vi "Periodic Tasks.vi"(8 "error in":errorcluster) -> ()   [LabVIEW 2012]
doc: "This VI runs in parallel to other tasks. It can contain as many user-defined periodic loops as you need. These can carry out PID or other sorts of timed response."
uses:
  <vilib>/Rock Robotics/SystemInterfaces/Utilities/FPGA_UtilitiesLED Source.ctl
  <vilib>/Rock Robotics/SystemInterfaces/Utilities/FPGA_UtilitiesLED State.ctl
  <vilib>/Rock Robotics/WPI/Compressor/WPI_CompressorGetSetRefNum.vi
  Robot Global Data.vi
panel:
  out "Shooter Speed":dbl
  out "Shooter Distance":dbl
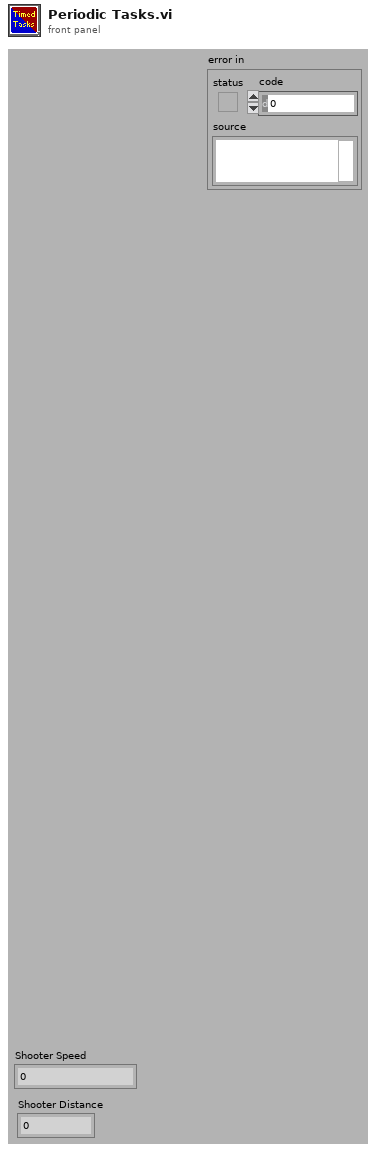
[diagram p1: front panel]
types:
  T1 = typedef "WPI_GyroDevRef.ctl" = cluster{"DevStatus":errorcluster, "Analog Module":T2, "Analog Channel":T3, "Offset":dbl, "Gain (VoltsPerDegree/Second)":dbl}
  T2 = typedef "FPGA_TypedefAnalogModule.ctl" = enum16{"Analog Module 1", "Analog Module 2"}
  T3 = typedef "FPGA_AIChannel.ctl" = enum8{"AI 1", "AI 2", "AI 3", "AI 4", "AI 5", "AI 6", "AI 7", "AI 8", "Invalid"}
  T4 = typedef "FPGA_UtilitiesLED State.ctl" = enum16{"Off", "On", "Toggle"}
  T5 = typedef "FPGA_UtilitiesLED Source.ctl" = enum16{"User LED", "FPGA LED"}
  T6 = typedef "WPI_DriverStationRobotMode2.ctl" = enum16{"Autonomous Disabled", "Autonomous Enabled", "Teleop Disabled", "Teleop Enabled", "Timeout", "Finish", "Test Disabled", "Test Enabled"}
  T7 = typedef "WPI_EncoderDevRef.ctl" = cluster{"DevStatus":errorcluster, "EncoderIndex":T8, "CounterIndex":T9, "DistancePerCount":dbl, "Decoding Type":T10}
  T8 = typedef "FPGA_EncoderIdx.ctl" = enum8{"Enc 0", "Enc 1", "Enc 2", "Enc 3", "Invalid"}
  T9 = typedef "FPGA_CounterCtrSystemIndex.ctl" = enum8{"Ctr 0", "Ctr 1", "Ctr 2", "Ctr 3", "Ctr 4", "Ctr 5", "Ctr 6", "Ctr 7", "Invalid"}
  T10 = typedef "WPI_EncoderType.ctl" = enum16{"1x", "2x", "4x"}
  T11 = enum16{"Off", "Close Pyramid 3pt", "Far Pyramid 3pt", "Feeder Shot", "UD Far 3pt Shot"}
  T12 = typedef "WPI_CompressorDevRef.ctl" = cluster{"DevStatus":errorcluster, "DigitalInputDevRef":T13, "RelayDevRef":T16}
  T13 = typedef "WPI_DigitalInputDevRef.ctl" = cluster{"DevStatus":errorcluster, "DIO Channel":T14, "Digital Module":T15}
  T14 = typedef "FPGA_DIOChannel.ctl" = enum8{"DIO 1", "DIO 2", "DIO 3", "DIO 4", "DIO 5", "DIO 6", "DIO 7", "DIO 8", "DIO 9", "DIO 10", "DIO 11", "DIO 12", "DIO 13", "DIO 14", "Invalid"}
  T15 = typedef "FPGA_TypedefDigitalModule.ctl" = enum16{"Digital Module 1", "Digital Module 2"}
  T16 = typedef "WPI_RelayDevRef.ctl" = cluster{"DevStatus":errorcluster, "Relay Channel":T17, "Digital Module":T15, "Relay Direction":T18}
  T17 = typedef "FPGA_DIORelayChannel.ctl" = enum8{"Relay 1", "Relay 2", "Relay 3", "Relay 4", "Relay 5", "Relay 6", "Relay 7", "Relay 8", "Invalid"}
  T18 = typedef "WPI_RelayDirection.ctl" = enum16{"Both directions", "Forward only", "Reverse only"}
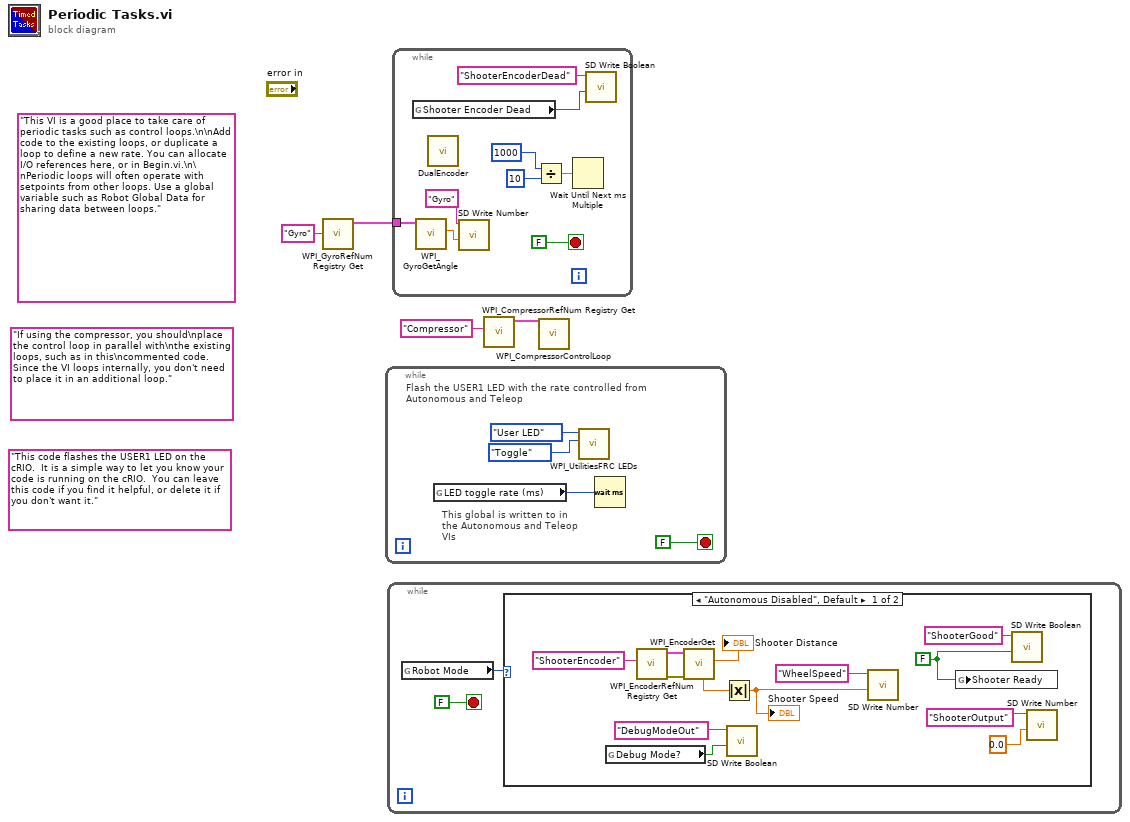
[diagram p0: block diagram]
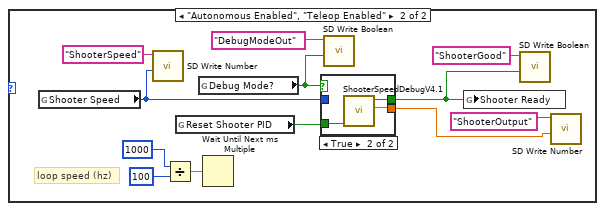
[diagram p2: hidden frame]
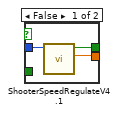
[diagram p3: hidden frame]
diagram:
  (unwired) "If using the compressor, you should\nplace the control loop in parallel with\nthe existing loops, such as in this\ncommented code. Since the VI loops internally, you don't need to place it in an additional loop."
  (unwired) "This code flashes the USER1 LED on the cRIO.  It is a simple way to let you know your code is running on the cRIO.  You can leave this code if you find it helpful, or delete it if you don't want it."
  (unwired) "This VI is a good place to take care of periodic tasks such as control loops.\n\nAdd code to the existing loops, or duplicate a loop to define a new rate. You can allocate I/O references here, or in Begin.vi.\n\nPeriodic loops will often operate with setpoints from other loops. Use a global variable such as Robot Global Data for sharing data between loops."
  n1 = call <vilib>:"WPI_GyroRefNum Registry Get.vi"("refnum name"="Gyro") -> ("GyroDevRef"=w3:T1)  [unwired: 9 in, 1 out]
  n2 = while {
    stop <- FALSE stop-if-true
    # "This global is written to in the Autonomous and Teleop VIs"
    # "Flash the USER1 LED with the rate controlled from Autonomous and Teleop"
    n3 = global read "Robot Global Data.vi" "LED toggle rate (ms)"() -> (w5:u32)
    n4 = call <vilib>:"WPI_UtilitiesFRC LEDs.vi"("State"=FPGA_UtilitiesLED_State."Toggle", "LED Type"=FPGA_UtilitiesLED_Source."User LED") -> ()  [unwired: 1 in, 9 out]
    n5 = Wait (ms)(milliseconds to wait=w5) -> ()  [unwired: 1 out]
  }
  n6 = while {
    stop <- FALSE stop-if-true
    n7 = global read "Robot Global Data.vi" "Robot Mode"() -> (w9:T6)
    n8 = case shown="\"Autonomous Disabled\", Default" w9 {
      frame "Autonomous Disabled", Default {
        w13 = FALSE ("Boolean")
        n9 = global read "Robot Global Data.vi" "Debug Mode?"() -> (w11:bool)
        n10 = call <vilib>:"WPI_EncoderRefNum Registry Get.vi"("refnum name"="ShooterEncoder") -> ("error out"=w21:errorcluster, "EncoderDevRef"=w22:T7)  [unwired: 9 in]
        n11 = call <vilib>:"WPI_EncoderGet.vi"("error in (no error)"=w21, "EncoderDevRef"=w22) -> ("Distance"=→"Shooter Distance":dbl, "Rate"=w20:dbl)  [unwired: 4 in, 4 out]
        n12 = Absolute Value(x=w20) -> (abs(x)=w18:dbl)
        "Shooter Speed" <- w18
        n13 = call <vilib>:"SD Write Boolean.vi"("Boolean"=w11, "Name"="DebugModeOut") -> ()  [unwired: 8 in, 2 out]
        n14 = call <vilib>:"SD Write Number.vi"("Numeric"=w18, "Name"="WheelSpeed") -> ()  [unwired: 8 in, 2 out]
        n15 = global write "Robot Global Data.vi" "Shooter Ready"(w13) -> ()
        n16 = call <vilib>:"SD Write Boolean.vi"("Boolean"=w13, "Name"="ShooterGood") -> ()  [unwired: 8 in, 2 out]
        n17 = call <vilib>:"SD Write Number.vi"("Numeric"=0.0, "Name"="ShooterOutput") -> ()  [unwired: 8 in, 2 out]
      }
      frame "Autonomous Enabled", "Teleop Enabled" {
        # "loop speed (hz)"
        n18 = global read "Robot Global Data.vi" "Shooter Speed"() -> (w31:T11)
        n19 = call <vilib>:"SD Write Number.vi"("Numeric"=w31, "Name"="ShooterSpeed") -> ()  [unwired: 8 in, 2 out]
        n20 = Divide(x=1000, y=100) -> (x/y=w33:dbl)
        n21 = global read "Robot Global Data.vi" "Reset Shooter PID"() -> (w26:bool)
        n22 = global read "Robot Global Data.vi" "Debug Mode?"() -> (w24:bool)
        n23 = Wait Until Next ms Multiple(millisecond multiple=w33) -> ()  [unwired: 1 out]
        n24 = case shown="True" w24 {
          tunnel: w31 -> [w38 _]
          tunnel: w26 -> [_ w41]
          tunnel: [w37 w40] -> w29
          tunnel: [w36 w39] -> w27
          frame False {
            n25 = call "ShooterSpeedRegulateV4.1.vi"("Shooter Speed"=w38) -> ("Voltage Output"=w36:dbl, "GO GO GO"=w37:bool)  [unwired: 9 in]
          }
          frame True {
            n26 = call "ShooterSpeedDebugV4.1.vi"("Reset PID"=w41) -> ("Wheel 1 Actual Voltage"=w39:dbl, "GO GO GO"=w40:bool)  [unwired: 9 in]
          }
        }
        n27 = call <vilib>:"SD Write Boolean.vi"("Boolean"=w24, "Name"="DebugModeOut") -> ()  [unwired: 8 in, 2 out]
        n28 = global write "Robot Global Data.vi" "Shooter Ready"(w29) -> ()
        n29 = call <vilib>:"SD Write Boolean.vi"("Boolean"=w29, "Name"="ShooterGood") -> ()  [unwired: 8 in, 2 out]
        n30 = call <vilib>:"SD Write Number.vi"("Numeric"=w27, "Name"="ShooterOutput") -> ()  [unwired: 8 in, 2 out]
      }
    }
  }
  n31 = while {
    tunnel: w3 -> [w49]
    stop <- FALSE stop-if-true
    n32 = global read "Robot Global Data.vi" "Shooter Encoder Dead"() -> (w42:bool)
    n33 = call <vilib>:"WPI_GyroGetAngle.vi"("GyroDevRef"=w49) -> ("Angle"=w48:dbl)  [unwired: 7 in, 3 out]
    n34 = call "DualEncoder.vi"() -> ()  [unwired: 7 in, 5 out]
    n35 = call <vilib>:"SD Write Number.vi"("Numeric"=w48, "Name"="Gyro") -> ()  [unwired: 8 in, 2 out]
    n36 = Divide(x=u32 1000 ("milliseconds to wait"), y=u32 10 ("milliseconds to wait")) -> (x/y=w46:dbl)
    n37 = Wait Until Next ms Multiple(millisecond multiple=w46) -> ()  [unwired: 1 out]
    n38 = call <vilib>:"SD Write Boolean.vi"("Boolean"=w42, "Name"="ShooterEncoderDead") -> ()  [unwired: 8 in, 2 out]
  }
  n39 = call <vilib>:"WPI_CompressorRefNum Registry Get.vi"("refnum name"="Compressor") -> ("CompressorDevRef"=w2:T12)  [unwired: 9 in, 1 out]
  n40 = call <vilib>:"WPI_CompressorControlLoop.vi"("CompressorDevRef"=w2) -> ()  [unwired: 11 in]
